vi "Create_Pos_array.vi"(2 "Traverse line":T1 {"Row Duration (mins)" format="%#.1f"; "Row No" min=0; "Trace Gas Concentration (%)" min=0.0 format="%#.2f"; "Emission Rate (l/min)" format="%#.2f"; "Tunnel Speed" format="%#.2f"; "Start X" format="%#.2f"; "Start Y" format="%#.2f"; "Start Z" format="%#.2f"; "End X" format="%#.2f"; "End Y" format="%#.2f"; "End Z" format="%#.2f"; "Averaging time (min)" min=0.0 format="%#.2f"}) -> (5 "Traverse line Out":T1 {"Row Duration (mins)" format="%#.1f"; "Row No" min=0; "Trace Gas Concentration (%)" min=0.0 format="%#.2f"; "Emission Rate (l/min)" format="%#.2f"; "Tunnel Speed" format="%#.2f"; "Start X" format="%#.2f"; "Start Y" format="%#.2f"; "Start Z" format="%#.2f"; "End X" format="%#.2f"; "End Y" format="%#.2f"; "End Z" format="%#.2f"; "Averaging time (min)" min=0.0 format="%#.2f"}, 6 "Error Messages":string, 7 "Array of Positions":dbl[][](array[numeric]) format="%.2f", 9 "Axis Traversed":enum16{"X traverse", "Y traverse", "Z traverse"}(ring))   [LabVIEW 2012]
uses:
  Traverse_cluster.ctl
  Spacing.ctl
  Controls/Multi_run_mode.ctl
  Globals/Extra_Commands_Global.vi
panel:
  # "X           Y            Z"
  # "Start"
  # "End"
  # "X           Y            Z"
  # "Start"
  # "End"
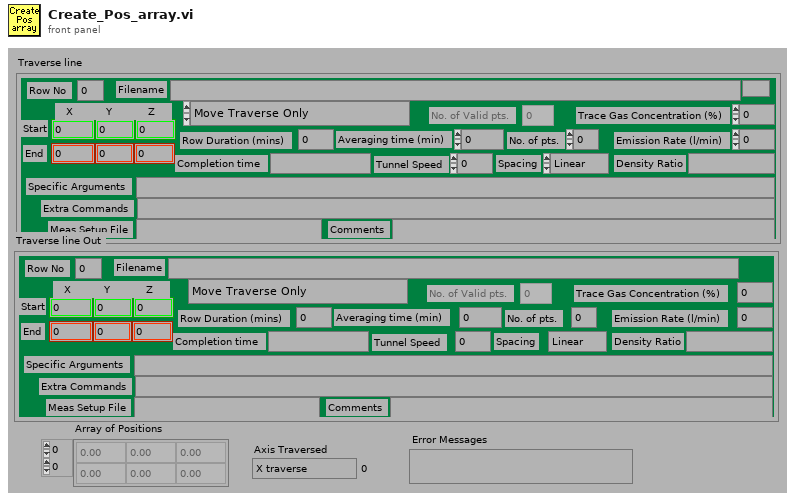
[diagram p1: front panel]
types:
  T1 = typedef "Traverse_cluster.ctl" = cluster{"Start X":dbl, "Start Y":dbl, "Start Z":dbl, "End X":dbl, "End Y":dbl, "End Z":dbl, "No. of pts.":i32, "Spacing":T2, "Filename":path, "Tunnel Speed":dbl, "Averaging time (min)":dbl, "Extra Commands":string, "Specific Arguments":string, "Emission Rate (l/min)":dbl, "Trace Gas Concentration (%)":dbl, "Density Ratio":string, "Comments":string, "Row No":i32, "Row Type Selector":T3, "Completion time":string, "Row Duration (mins)":dbl, "No. of Valid pts.":i32, "Meas Setup File":string}
  T2 = typedef "Spacing.ctl" = enum16{"Linear", "Log", "Gauss", "Specified", "N/A"}
  T3 = typedef "Multi_run_mode.ctl" = enum16{"Move Traverse Only", "Set Tunnel Speed Only", "Set Source Only", "Set Measurement Conditions", "Single Measurement", "Vertical Profile", "Lateral Profile", "Longitudinal Profile", "Explore Volume", "Multi-Axis Profile", "Auto Calibrate", "Meas Fast FID Bkgnd", "Check Beam Power", "Scanning Valve Measurement", "Run VI Named:", "Set ADAM Ch", "Wait (minutes)", "Send Message", "Synchronize With:", "Fall Back to this Row", "Turn Off Row Repeating", "Blank Row", "Traverse 3D Volume"}
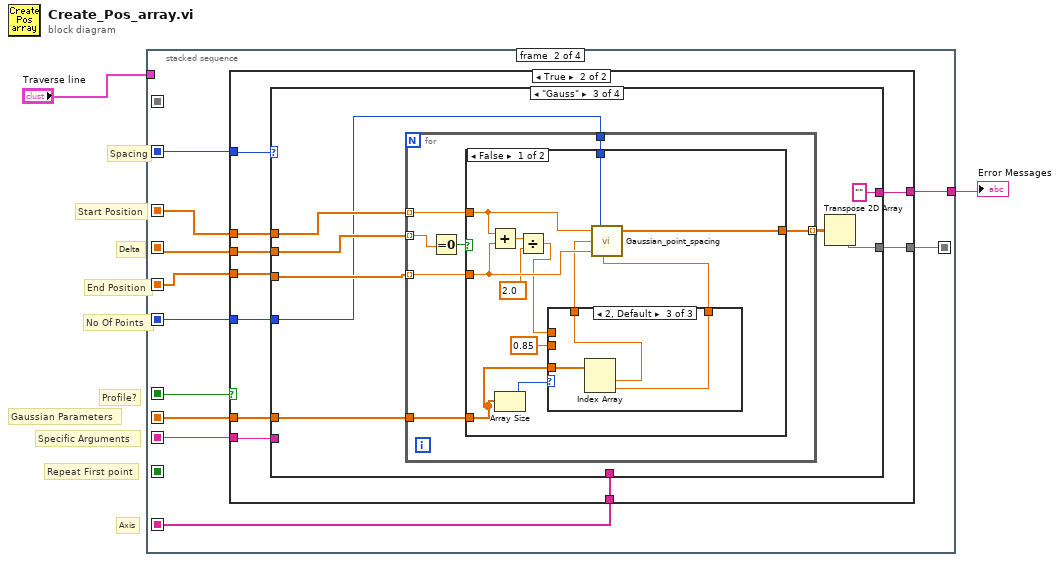
[diagram p0: block diagram]
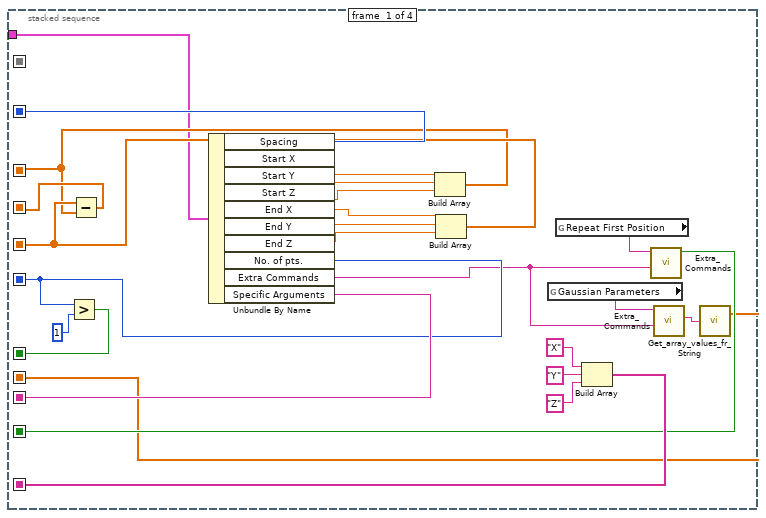
[diagram p2: hidden frame]
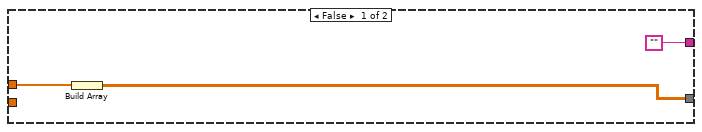
[diagram p3: hidden frame]
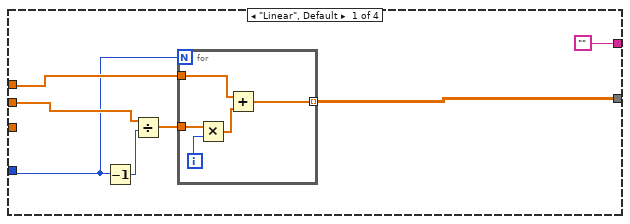
[diagram p4: hidden frame]
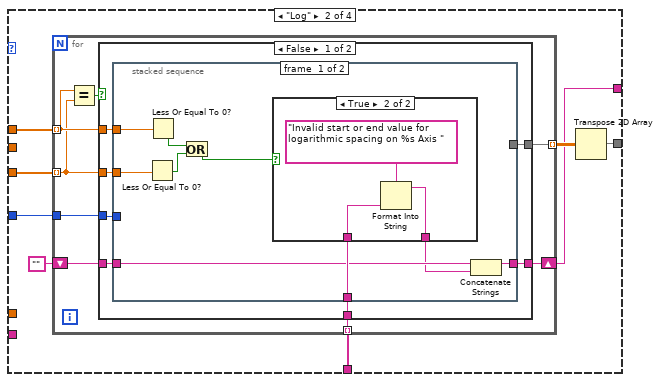
[diagram p5: hidden frame]
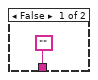
[diagram p6: hidden frame]
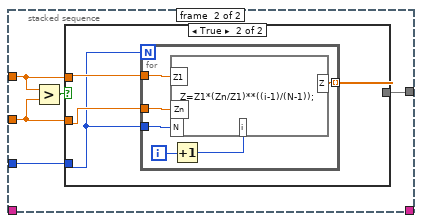
[diagram p7: hidden frame]
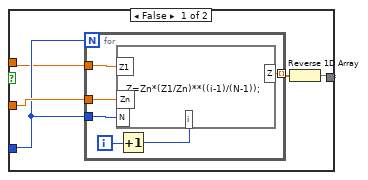
[diagram p8: hidden frame]
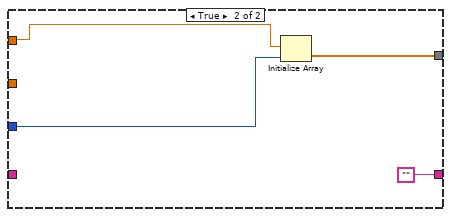
[diagram p9: hidden frame]
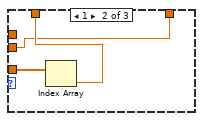
[diagram p11: hidden frame]
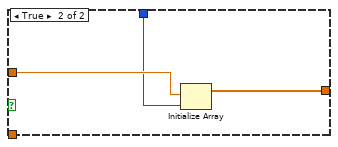
[diagram p12: hidden frame]
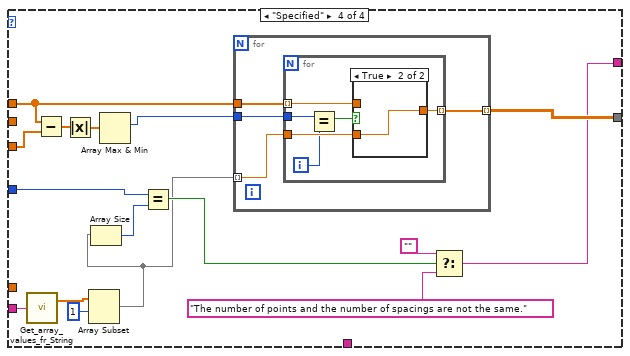
[diagram p13: hidden frame]
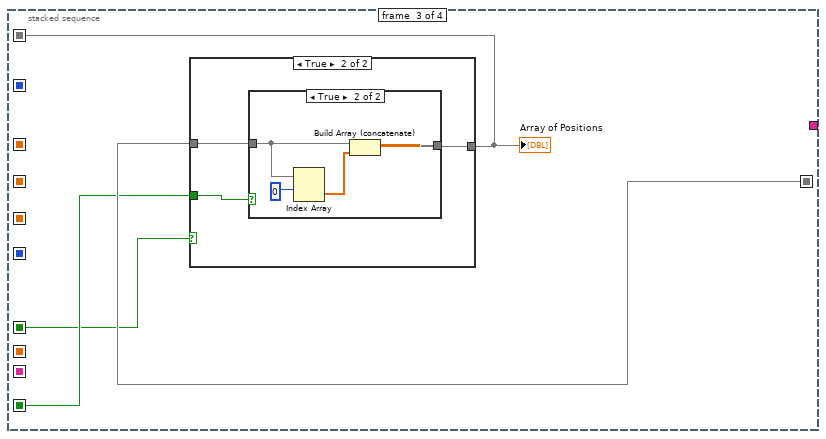
[diagram p15: hidden frame]
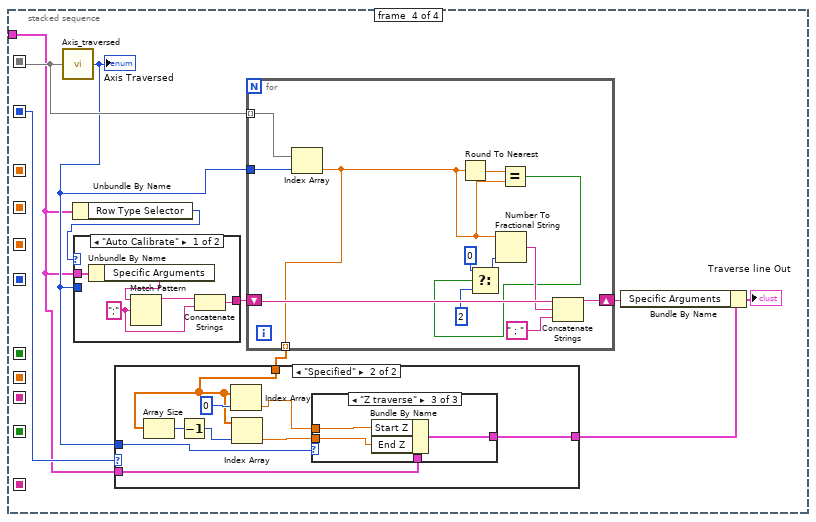
[diagram p18: hidden frame]
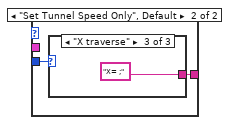
[diagram p19: hidden frame]
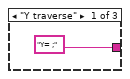
[diagram p20: hidden frame]
diagram:
  # "Gaussian Parameters"
  # "Axis"
  # "Profile?"
  # "Delta"
  # "Repeat First point"
  # "Spacing"
  # "No Of Points"
  # "Specific Arguments"
  # "End Position"
  # "Start Position"
  n1 = stacked-sequence {
    seq-local: [_ w38 _ _] -> [_ _ w199 _]
    seq-local: [w14 _ _ _] -> [_ w35 _ _]
    seq-local: [w19 _ _ _] -> [_ w33 _ _]
    seq-local: [w20 _ _ _] -> [_ w34 _ _]
    seq-local: [w16 _ _ _] -> [_ w31 _ _]
    seq-local: [w18 _ _ _] -> [_ w37 _ _]
    seq-local: [w27 _ _ _] -> [_ w36 _ w214]
    seq-local: [w8 _ _ _] -> [_ _ w198 _]
    seq-local: [w15 _ _ _] -> [_ w30 w197 _]
    seq-local: [w10 _ _ _] -> [_ w29 _ _]
    seq-local: [_ _ w196 _] -> [_ _ _ w218]
    seq-local: [w3 _ _ _] -> [_ w28 _ _]
    tunnel: [_ w32 _ _] -> w2
    tunnel: "Traverse line" -> [w7 _ _ w209]
    frame #0 {
      n2 = Unbundle By Name(w7) -> ("Spacing"=w27:T2, "Start X"=w26:dbl, "Start Y"=w25:dbl, "Start Z"=w24:dbl, "End X"=w23:dbl, "End Y"=w22:dbl, "End Z"=w21:dbl, "No. of pts."=w16:i32, "Extra Commands"=w5:string, "Specific Arguments"=w18:string)
      n3 = Greater?(x=w16, y=1) -> (0:w15:bool)
      n4 = Build Array(w26, w25, w24) -> (w14:dbl[])
      n5 = Build Array(w23, w22, w21) -> (w20:dbl[])
      n6 = Subtract(x=w20, y=w14) -> (x-y=w19:dbl[])
      n7 = global read "Extra_Commands_Global.vi" "Gaussian Parameters"() -> (w6:string)
      n8 = global read "Extra_Commands_Global.vi" "Repeat First Position"() -> (w9:string)
      n9 = Build Array("X", "Y", "Z") -> (w10:string[])
      n10 = call "Extra_Commands.vi"("String to Search"=w5, "Command"=w9) -> ("Command Found"=w8:bool)  [unwired: 1 in, 4 out]
      n11 = call "Extra_Commands.vi"("String to Search"=w5, "Command"=w6) -> ("String Value"=w4:string)  [unwired: 1 in, 4 out]
      n12 = call "Get_array_values_fr_String.vi"("String Value"=w4) -> ("Numeric Array"=w3:dbl[])  [unwired: 1 out]
    }
    frame #1 {
      n13 = case shown="True" w30 {
        tunnel: [w40 w51] -> w38
        tunnel: w37 -> [_ w50]
        tunnel: w36 -> [_ w49]
        tunnel: w35 -> [w41 w48]
        tunnel: w34 -> [_ w47]
        tunnel: w33 -> [_ w46]
        tunnel: w31 -> [_ w45]
        tunnel: ["" w44] -> w32
        tunnel: w29 -> [_ w43]
        tunnel: w28 -> [_ w42]
        frame False {
          n14 = Build Array(w41) -> (w40:dbl[][])
        }
        frame True {
          n15 = case shown="\"Gauss\"" w49 {
            tunnel: w47 -> [_ w69 w135 w175]
            tunnel: w48 -> [w57 w70 w136 w171]
            tunnel: w45 -> [w55 w71 w134 w180]
            tunnel: [w58 w68 w133 w182] -> w51
            tunnel: w46 -> [w56 _ w137 _]
            tunnel: w50 -> [_ _ _ w183]
            tunnel: ["" w64 "" ("f") w176] -> w44
            tunnel: w43 -> [_ w66 _ _]
            tunnel: w42 -> [_ _ w130 _]
            frame "Linear", Default {
              n16 = Decrement(x=w55) -> (x-1=w53:i32)
              n17 = Divide(x=w56, y=w53) -> (x/y=w54:dbl[])
              n18 = for {
                N: w55 -> [_]
                tunnel: w54 -> [w62]
                tunnel: w57 -> [w60]
                tunnel: [w59] -> w58 mode=indexing
                i -> [w63]
                n19 = Multiply(x=w62, y=w63) -> (x*y=w61:dbl[])
                n20 = Add(x=w60, y=w61) -> (x+y=w59:dbl[])
              }
            }
            frame "Log" {
              n21 = for {
                tunnel: [w79] -> w67 mode=indexing
                tunnel: w70 -> [w77] mode=indexing
                tunnel: w69 -> [w76] mode=indexing
                tunnel: w71 -> [w78]
                tunnel: w66 -> [w74] mode=indexing
                shift-right: [w72] -> w64
                shift-left: "" -> [w73]
                n22 = Equal?(x=w77, y=w76) -> (x = y?=w75:bool)
                n23 = case shown="False" w75 {
                  tunnel: w78 -> [w86 w128]
                  tunnel: w76 -> [w85 _]
                  tunnel: w77 -> [w84 w127]
                  tunnel: [w83 w129] -> w79
                  tunnel: w74 -> [w82 _]
                  tunnel: w73 -> [w81 _]
                  tunnel: [w80 ""] -> w72
                  frame False {
                    n24 = stacked-sequence {
                      tunnel: [_ w103] -> w83
                      tunnel: w84 -> [w95 w102]
                      tunnel: w85 -> [w94 w101]
                      tunnel: w86 -> [_ w100]
                      tunnel: w82 -> [w90 _]
                      tunnel: w81 -> [w89 _]
                      tunnel: [w87 _] -> w80
                      frame #0 {
                        n25 = Less Or Equal To 0?(x=w94) -> (x <= 0?=w93:bool)
                        n26 = Less Or Equal To 0?(x=w95) -> (x <= 0?=w92:bool)
                        n27 = Or(x=w92, y=w93) -> (x .or. y?=w91:bool)
                        n28 = case shown="True" w91 {
                          tunnel: w90 -> [_ w99]
                          tunnel: ["" w97] -> w88
                          frame False {
                          }
                          frame True {
                            n29 = Format Into String(format string="Invalid start or end value for logarithmic spacing on %s Axis " ("Format String"), w99) -> (resulting string=w97:string)  [unwired: 2 in, 1 out]
                          }
                        }
                        n30 = Concatenate Strings(w89, w88) -> (w87:string)
                      }
                      frame #1 {
                        n31 = Greater?(x=w102, y=w101) -> (0:w104:bool)
                        n32 = case shown="True" w104 {
                          tunnel: [w106 w116] -> w103
                          tunnel: w102 -> [w105 w119]
                          tunnel: w101 -> [w109 w118]
                          tunnel: w100 -> [w108 w117]
                          frame False {
                            n33 = for {
                              N: w108 -> [_]
                              tunnel: w109 -> [w112]
                              tunnel: w108 -> [w111]
                              tunnel: [w113] -> w107 mode=indexing
                              tunnel: w105 -> [w110]
                              i -> [w115]
                              n34 = Increment(x=w115) -> (x+1=w114:i32)
                              n35 = formula code="Z=Zn*(Z1/Zn)**((i-1)/(N-1));"("i"=w114, "N"=w111, "Zn"=w112, "Z1"=w110) -> ("Z"=w113:dbl)
                            }
                            n36 = Reverse 1D Array(array=w107) -> (reversed array=w106:dbl[])
                          }
                          frame True {
                            n37 = for {
                              N: w117 -> [_]
                              tunnel: w119 -> [w125]
                              tunnel: w118 -> [w124]
                              tunnel: w117 -> [w121]
                              tunnel: [w120] -> w116 mode=indexing
                              i -> [w123]
                              n38 = Increment(x=w123) -> (x+1=w122:i32)
                              n39 = formula code="Z=Z1*(Zn/Z1)**((i-1)/(N-1));"("i"=w122, "N"=w121, "Zn"=w124, "Z1"=w125) -> ("Z"=w120:dbl)
                            }
                          }
                        }
                      }
                    }
                  }
                  frame True {
                    n40 = Initialize Array(w127, w128) -> (w129:dbl[])
                  }
                }
              }
              n41 = Transpose 2D Array(2D array=w67) -> (transposed array=w68:dbl[][])
            }
            frame "Gauss" {
              n42 = for {
                tunnel: w137 -> [w139] mode=indexing
                tunnel: w136 -> [w143] mode=indexing
                tunnel: w135 -> [w142] mode=indexing
                tunnel: w134 -> [w141]
                tunnel: [w140] -> w132 mode=indexing
                tunnel: w130 -> [w138]
                n43 = Equal To 0?(x=w139) -> (x = 0?=w144:bool)
                n44 = case shown="False" w144 {
                  tunnel: w143 -> [w154 w167]
                  tunnel: w142 -> [w153 _]
                  tunnel: w141 -> [w156 w166]
                  tunnel: [w155 w165] -> w140
                  tunnel: w138 -> [w146 _]
                  frame False {
                    n45 = Add(x=w154, y=w153) -> (x+y=w152:dbl)
                    n46 = Array Size(array=w146) -> (size(s)=w150:i32)
                    n47 = Divide(x=w152, y=2.0) -> (x/y=w148:dbl)
                    n48 = case shown="2, Default" w150 {
                      tunnel: [w158 w160 w163] -> w149
                      tunnel: w148 -> [w158 _ _]
                      tunnel: [w157 w159 w162] -> w147
                      tunnel: w146 -> [_ w161 w164]
                      tunnel: 0.85 ("Guass intensity") -> [w157 w159 _]
                      frame 0 {
                      }
                      frame 1 {
                        n49 = Index Array(array=w161) -> (element=w160:dbl)  [unwired: 1 in]
                      }
                      frame 2, Default {
                        n50 = Index Array(array=w164) -> (element #1=w163:dbl, element #2=w162:dbl)  [unwired: 2 in]
                      }
                    }
                    n51 = call "Gaussian_point_spacing.vi"("Start point"=w154, "No of points"=w156, "Centre point"=w149, "End point"=w153, "Guass intensity"=w147) -> ("Positions"=w155:dbl[])  [unwired: 2 out]
                  }
                  frame True {
                    n52 = Initialize Array(w167, w166) -> (w165:dbl[])
                  }
                }
              }
              n53 = Transpose 2D Array(2D array=w132) -> (transposed array=w133:dbl[][])
            }
            frame "Specified" {
              n54 = call "Get_array_values_fr_String.vi"("String Value"=w183) -> ("Numeric Array"=w170:dbl[])  [unwired: 1 out]
              n55 = Subtract(x=w171, y=w175) -> (x-y=w174:dbl[])
              n56 = Absolute Value(x=w174) -> (abs(x)=w173:dbl[])
              n57 = Array Subset(array=w170, index=1) -> (w168:dbl[])  [unwired: 1 in]
              n58 = Array Size(array=w168) -> (size(s)=w181:i32)
              n59 = Array Max & Min(array=w173) -> (max index (indices)=w172:i32)  [unwired: 3 out]
              n60 = Equal?(x=w180, y=w181) -> (x = y?=w179:bool)
              n61 = for {
                tunnel: w168 -> [w185] mode=indexing
                tunnel: [w186] -> w182 mode=indexing
                tunnel: w172 -> [w187]
                tunnel: w171 -> [w184]
                n62 = for {
                  tunnel: w187 -> [w191]
                  tunnel: [w193] -> w186 mode=indexing
                  tunnel: w185 -> [w192]
                  tunnel: w184 -> [w188] mode=indexing
                  i -> [w190]
                  n63 = Equal?(x=w191, y=w190) -> (x = y?=w189:bool)
                  n64 = case shown="True" w189 {
                    tunnel: [w194 w195] -> w193
                    tunnel: w192 -> [_ w195]
                    tunnel: w188 -> [w194 _]
                    frame False {
                    }
                    frame True {
                    }
                  }
                }
              }
              n65 = Select(t="", s=w179, f="The number of points and the number of spacings are not the same.") -> (s? t:f=w176:string)
            }
          }
        }
      }
    }
    frame #2 {
      n66 = case shown="True" w197 {
        tunnel: [w200 w203] -> w196
        tunnel: w199 -> [w200 w202]
        tunnel: w198 -> [_ w201]
        frame False {
        }
        frame True {
          n67 = case shown="True" w201 {
            tunnel: [w204 w208] -> w203
            tunnel: w202 -> [w204 w206]
            frame False {
            }
            frame True {
              n68 = Index Array(array=w206, index (row)=0) -> (element=w207:dbl[])  [unwired: 1 in]
              n69 = Build Array (concatenate)(w206, w207) -> (w208:dbl[][])
            }
          }
        }
      }
      "Array of Positions" <- w196
    }
    frame #3 {
      n70 = call "Axis_traversed.vi"("Position array"=w218) -> ("Axis Traversed"=w212:enum16{"X traverse", "Y traverse", "Z traverse"})  [unwired: 4 out]
      "Axis Traversed" <- w212
      n71 = Unbundle By Name(w209) -> ("Row Type Selector"=w210:T3)
      n72 = case shown="\"Auto Calibrate\"" w210 {
        tunnel: [w221 w225] -> w215
        tunnel: w212 -> [_ w224]
        tunnel: w209 -> [w223 _]
        frame "Auto Calibrate" {
          w219 = ";" ("regular expression")
          n73 = Unbundle By Name(w223) -> ("Specific Arguments"=w222:string)
          n74 = Match Pattern(string=w222, regular expression=w219) -> (before substring=w220:string)  [unwired: 4 out]
          n75 = Concatenate Strings(w220, w219) -> (w221:string)
        }
        frame "Set Tunnel Speed Only", Default {
          n76 = case shown="\"X traverse\"" w224 {
            tunnel: ["Y= ;" "Z= ;" "X= ;"] -> w225
            frame "Y traverse" {
            }
            frame "Z traverse" {
            }
            frame "X traverse" {
            }
          }
        }
      }
      n77 = for {
        tunnel: w212 -> [w262]
        tunnel: w218 -> [w252] mode=indexing
        shift-right: [w260] -> w217
        shift-left: w215 -> [w261]
        tunnel: [w251] -> w213 mode=indexing
        n78 = Index Array(array=w252, index=w262) -> (element=w251:dbl)
        n79 = Round To Nearest(number=w251) -> (nearest integer value=w254:dbl)
        n80 = Equal?(x=w254, y=w251) -> (x = y?=w253:bool)
        n81 = Select(t=0, s=w253, f=2) -> (s? t:f=w257:i32)
        n82 = Number To Fractional String(number=w251, precision (6)=w257) -> (F-format string=w259:string)  [unwired: 2 out]
        n83 = Concatenate Strings(w261, w259, " ; " ("string")) -> (w260:string)
      }
      n84 = case shown="\"Specified\"" w214 {
        tunnel: w213 -> [_ w233]
        tunnel: w212 -> [_ w238]
        tunnel: w209 -> [w229 w237]
        tunnel: [w229 w232] -> w211
        frame "Linear", Default {
        }
        frame "Specified" {
          n85 = Array Size(array=w233) -> (size(s)=w236:i32)
          n86 = Decrement(x=w236) -> (x-1=w234:i32)
          n87 = Index Array(array=w233, index=0) -> (element=w231:dbl)
          n88 = Index Array(array=w233, index=w234) -> (element=w230:dbl)
          n89 = case shown="\"Z traverse\"" w238 {
            tunnel: w237 -> [w242 w246 w250]
            tunnel: [w241 w245 w249] -> w232
            tunnel: w231 -> [w240 w244 w248]
            tunnel: w230 -> [w239 w243 w247]
            frame "X traverse" {
              n90 = Bundle By Name(cluster=w242, "Start X"=w240, "End X"=w239) -> (w241:T1)
            }
            frame "Y traverse" {
              n91 = Bundle By Name(cluster=w246, "Start Y"=w244, "End Y"=w243) -> (w245:T1)
            }
            frame "Z traverse" {
              n92 = Bundle By Name(cluster=w250, "Start Z"=w248, "End Z"=w247) -> (w249:T1)
            }
          }
        }
      }
      n93 = Bundle By Name(cluster=w211, "Specific Arguments"=w217) -> (→"Traverse line Out":T1)
    }
  }
  "Error Messages" <- w2
